vi "Get Handled Errors In Display Order.vi"(1 "Display Order":T3, 2 "Handled Errors (chronological order)":T1[](array[typedef])) -> (0 "Handled Errors (display order)":T1[](array[typedef]))   [LabVIEW 2023, in "Error Manager.lvlib"]
doc: "This VI outputs the array of handled errors in the \"display order\". This means that the output array of Handled Errors uses the same ordering as the MCL value (array of I32)."
uses:
  Error Manager.lvlib
  Handled Error (cluster).ctl
  Read-Unread Status (enum).ctl
  Display Order (enum).ctl
panel:
  # "Development\nControls or indicators that are useful for development or testing, but which are not outputs of the VI."
  # "Input\nInputs to the VI"
  # "Output\nOutputs of the VI"
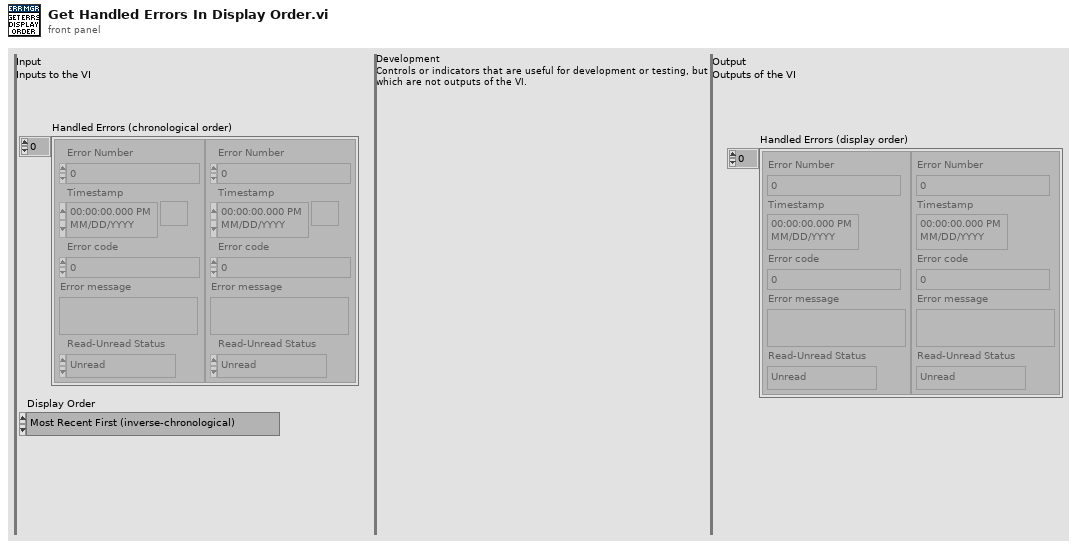
[diagram p1: front panel]
types:
  T1 = typedef "Error Manager.lvlib/Handled Error (cluster).ctl" = cluster{"Error Number":i32, "Timestamp":timestamp, "Error code":i32, "Error message":string, "Read-Unread Status":T2}
  T2 = typedef "Error Manager.lvlib/Read-Unread Status (enum).ctl" = enum16{"Unread", "Read"}
  T3 = typedef "Error Manager.lvlib/Display Order (enum).ctl" = enum16{"Most Recent First (inverse-chronological)", "Oldest First (chronological)"}
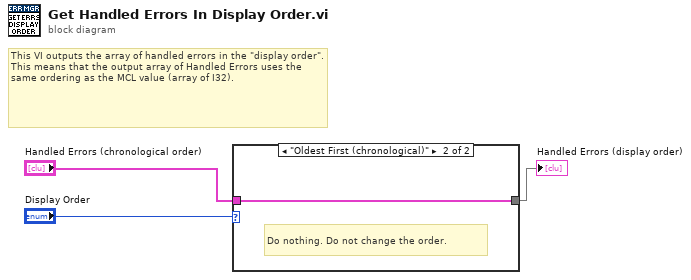
[diagram p0: block diagram]
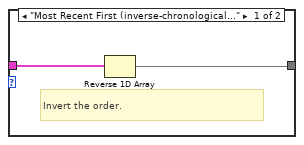
[diagram p2: hidden frame]
diagram:
  # "This VI outputs the array of handled errors in the \"display order\". This means that the output array of Handled Errors uses the same ordering as the MCL value (array of I32)."
  n1 = case shown="\"Oldest First (chronological)\"" "Display Order" {
    tunnel: "Handled Errors (chronological order)" -> [w5 w6]
    tunnel: [w4 w6] -> w1
    frame "Most Recent First (inverse-chronological)" {
      # "Invert the order."
      n2 = Reverse 1D Array(array=w5) -> (reversed array=w4:T1[])
    }
    frame "Oldest First (chronological)" {
      # "Do nothing. Do not change the order."
    }
  }
  "Handled Errors (display order)" <- w1
